vi "AppConfigXMLToType.vi"(8 "error in (no error)":errorcluster, 10 "Config in":variant, 11 "LSEPlugin in":refnum<class "LSEPlugin.lvclass">) -> (0 "error out":errorcluster, 3 "LSEPlugin out":refnum<class "LSEPlugin.lvclass">)   [LabVIEW 2014, in "AppPlugins.lvlib" / "LSEPlugin.lvclass"]
uses:
  LSEPlugin.lvclass
  PublicAPI/Typedefs/LSEConfig.ctl
  LSEPlugin.lvclass/LSEPlugin.ctl
  Accessors/Write LSEConfig.vi
  <vilib>/Utility/error.llb/Error Cluster From Error Code.vi
  <vilib>/ErrorRing/Error Ring.xnode
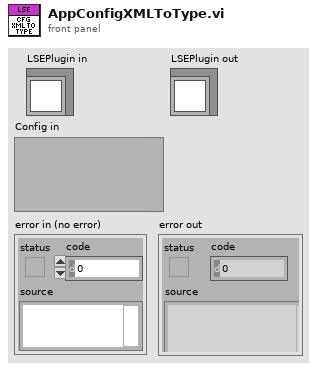
[diagram p1: front panel]
types:
  T1 = typedef "AppPlugins.lvlib/LSEPlugin.lvclass/LSEConfig.ctl" = cluster{"NoiseVariance":dbl, "IEEESystem":u32, "PMULocations":u32[], "Vindex":i32, "Iindex":i32, "DynamicRef":string}
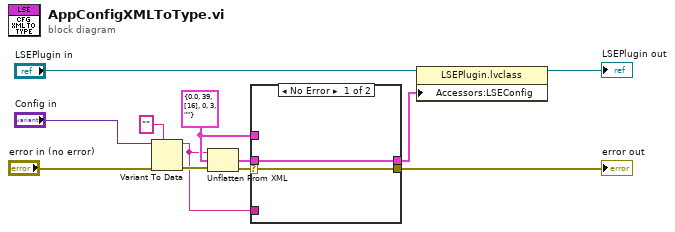
[diagram p0: block diagram]
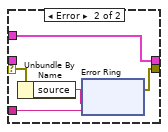
[diagram p2: hidden frame]
diagram:
  w2 = T1 {"NoiseVariance"=0.0, "IEEESystem"=39, "PMULocations"=[16], "Vindex"=0, "Iindex"=3, "DynamicRef"=""} ("LSEConfig")
  n1 = Variant To Data(error in="error in (no error)", type="", Variant="Config in") -> (data=w1:string, error out=w7:errorcluster)
  n2 = Unflatten From XML(xml string=w1, type=w2, error in (no error)=w7) -> (value=w5:T1, error out=w6:errorcluster)
  n3 = case shown="No Error" w6 {
    selector: w6 -> [w13 w18]
    tunnel: w5 -> [w14 _]
    tunnel: [w14 w19] -> w4
    tunnel: [w13 w15] -> w3
    tunnel: w2 -> [_ w19]
    tunnel: w1 -> [_ w16]
    frame No Error {
    }
    frame Error {
      n4 = Unbundle By Name(w18) -> ("source"=w17:string)
      n5 = xnode "Error Ring"("parameter 0"=w17, "parameter 1"=w16) -> ("error out"=w15:errorcluster)
    }
  }
  "error out" <- w3
  n6 = property class="LSEPlugin.lvclass"(reference="LSEPlugin in", "Accessors:LSEConfig"=w4) -> (reference out=→"LSEPlugin out":refnum<class "LSEPlugin.lvclass">)  [unwired: 1 in, 1 out]
